vi "Status.vi"(8 "error in (no error)":errorcluster, 11 "SimPump in":refnum<class "SimPump.lvclass">) -> (0 "error out":errorcluster, 1 "state":bool, 2 "volume pumped":dbl, 3 "SimPump out":refnum<class "SimPump.lvclass">)   [LabVIEW 2019, in "SimPump.lvclass"]
doc: "Returns the status of the pump such as the state and the volume pumped.\n\nwww.sciware.com.au"
uses:
  SimPump.lvclass
  SimPump.lvclass/SimPump.ctl
panel:
  # "BSD License (http://www.opensource.org/licenses/bsd-license.php)"
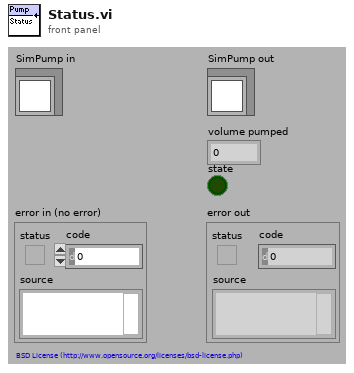
[diagram p1: front panel]
types:
  T1 = typedef "SimPump.lvclass/DataRef.ctl" = refnum<data-value>
  T2 = typedef "SimPump.lvclass/DataMembers.ctl" = cluster{"flow rate":dbl, "volume to pump":dbl, "state":bool, "ti":u32, "t0":u32}
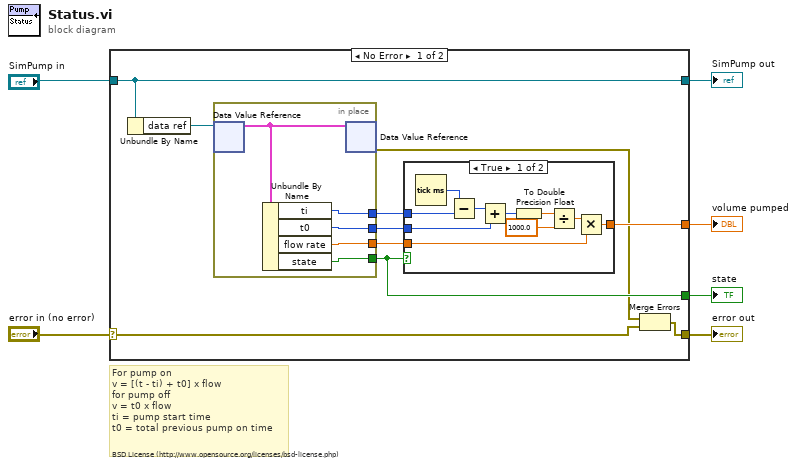
[diagram p0: block diagram]
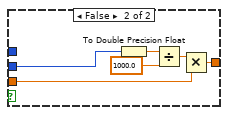
[diagram p2: hidden frame]
diagram:
  # "BSD License (http://www.opensource.org/licenses/bsd-license.php)"
  # "For pump on\nv = [(t - ti) + t0] x flow\nfor pump off\nv = t0 x flow\nti = pump start time\nt0 = total previous pump on time"
  n1 = case shown="No Error" "error in (no error)" {
    selector: "error in (no error)" -> [w7 w39]
    tunnel: [w10 w39] -> w4
    tunnel: [w16 w38] -> w3
    tunnel: "SimPump in" -> [w16 w38]
    tunnel: [w12 _] -> w2
    tunnel: [w11 _] -> w1
    frame No Error {
      n2 = Unbundle By Name(w16) -> ("data ref"=w8:T1)
      n3 = in-place {
        in-place-border: [w36] -> w11
        in-place-border: [w35] -> w15
        in-place-border: [w34] -> w14
        in-place-border: [w33] -> w13
        n4 = in-place-dvr #1(w8) -> (w37:T2)  [unwired: 1 out]
        n5 = Unbundle By Name(w37) -> ("ti"=w35:u32, "t0"=w34:u32, "flow rate"=w33:dbl, "state"=w36:bool)
        n6 = in-place-dvr #1(w37) -> (w9:errorcluster)  [unwired: 1 out]
      }
      n7 = case shown="True" w11 {
        tunnel: w15 -> [w26 _]
        tunnel: w14 -> [w23 w27]
        tunnel: w13 -> [w18 w29]
        tunnel: [w17 w28] -> w12
        frame True {
          n8 = Tick Count (ms)() -> (millisecond timer value=w25:u32)
          n9 = Subtract(x=w25, y=w26) -> (x-y=w24:u32)
          n10 = Add(x=w24, y=w23) -> (x+y=w22:u32)
          n11 = To Double Precision Float(number=w22) -> (double precision float=w21:dbl)
          n12 = Divide(x=w21, y=1000.0) -> (x/y=w19:dbl)
          n13 = Multiply(x=w19, y=w18) -> (x*y=w17:dbl)
        }
        frame False {
          n14 = To Double Precision Float(number=w27) -> (double precision float=w32:dbl)
          n15 = Divide(x=w32, y=1000.0) -> (x/y=w30:dbl)
          n16 = Multiply(x=w30, y=w29) -> (x*y=w28:dbl)
        }
      }
      n17 = Merge Errors(w9, w7) -> (w10:errorcluster)
    }
    frame Error {
    }
  }
  "error out" <- w4
  "SimPump out" <- w3
  "volume pumped" <- w2
  "state" <- w1
